vi "CreateEvents.vi"(8 "error in (no error)":errorcluster, 11 "TestApplication in":refnum<class "TestApplication.lvclass">) -> (0 "error out":errorcluster, 3 "TestApplication out":refnum<class "TestApplication.lvclass">)   [LabVIEW 2022 SP3, in "Demo.lvlib" / "TestApplication.lvclass"]
uses:
  TestApplication.lvclass
  _Events.ctl
  TestApplication.lvclass/TestApplication.ctl
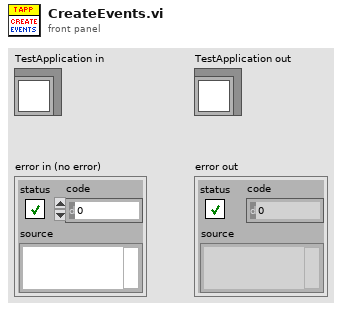
[diagram p1: front panel]
types:
  T1 = typedef "Demo.lvlib/TestApplication.lvclass/_Events.ctl" = cluster{"ToggleLed":refnum<user-event>}
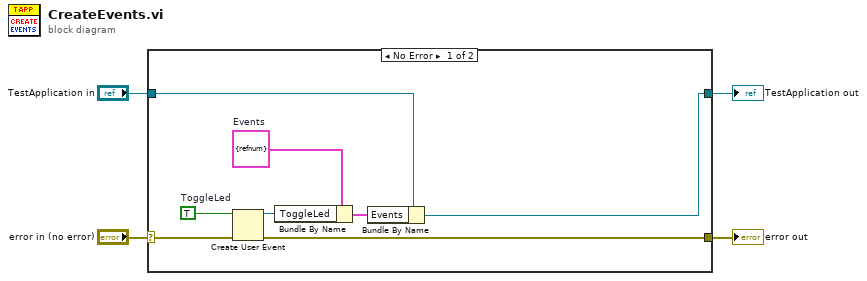
[diagram p0: block diagram]
diagram:
  n1 = case shown="No Error" "error in (no error)" {
    selector: "error in (no error)" -> [w11 w14]
    tunnel: [w10 w14] -> w3
    tunnel: [w6 w13] -> w1
    tunnel: "TestApplication in" -> [w5 w13]
    frame No Error {
      w9 = T1 {"ToggleLed"=refnum}  # Events
      w12 = TRUE  # ToggleLed
      n2 = Create User Event(user event datatype=w12, error in=w11) -> (user event=w8:refnum<user-event>, error out=w10:errorcluster)
      n3 = Bundle By Name(cluster=w9, "ToggleLed"=w8) -> (w7:T1)
      n4 = Bundle By Name(cluster=w5, "Events"=w7) -> (w6:refnum<class "TestApplication.lvclass">)
    }
    frame Error {
    }
  }
  "error out" <- w3
  "TestApplication out" <- w1
